vi "Autonomous Independent.vi"() -> ()   [LabVIEW 2013]
doc: "This VI is called when autonomous begins, and will automatically be terminated when autonomous ends. You can carry out timed or sensor driven robot movement independently without needing to return to the caller."
uses:
  <vilib>/Rock Robotics/WPI/Solenoid/WPI_SolenoidValue.ctl
  Robot Global Data.vi
  <vilib>/Rock Robotics/WPI/Solenoid/WPI_SolenoidSetEnum.vi
  <vilib>/Rock Robotics/WPI/RobotDrive/WPI_RobotDriveArcadeDrive_Standard(NoSaturation).vi
  <vilib>/Rock Robotics/WPI/RobotDrive/WPI_RobotDriveGetSetRefNum.vi
  <vilib>/Rock Robotics/WPI/Joystick/WPI_JoystickGetSetRefNum.vi
panel:
  out "Motor Values":dbl[](array[numeric])
  in  "Current Shooter Status":T1(ring)
  out "Timer for firing mech 2":dbl
  out "Timer for firing mech":dbl
  out "Hot?":bool
  out "Current Movement, for debugging":T2 {"Y Joystick Value" scale=1.0..-1.0; "X Joystick Value" scale=-1.0..1.0}
  in  "Array of robot movements":T3(array[cluster]) {"Y Joystick Value" scale=1.0..-1.0; "X Joystick Value" scale=-1.0..1.0}
  # "Be sure to right-click and choose Data Operations>>Make Current Value default if you want to save the array values with the VI"
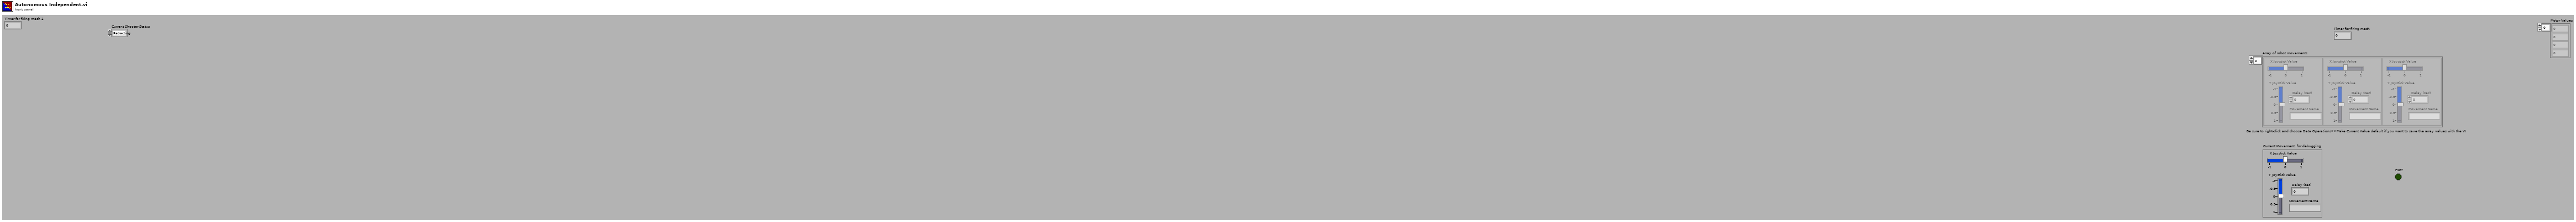
[diagram p1: front panel]
types:
  T1 = enum16{"Retracting", "Firing", "Ready to fire", "Pulling back", "Just fired"}
  T2 = cluster{"X Joystick Value":dbl, "Y Joystick Value":dbl, "Delay (sec)":dbl, "Movement Name":string}
  T3 = cluster{"X Joystick Value":dbl, "Y Joystick Value":dbl, "Delay (sec)":dbl, "Movement Name":string}[]
  T4 = typedef "WPI_JoystickDevRef.ctl" = cluster{"Device":T5}
  T5 = typedef "WPI_JoystickDeviceEnum.ctl" = enum16{"USB 1", "USB 2", "USB 3", "USB 4", "Kinect 1", "Kinect 2"}
  T6 = cluster{"axis 1 (x)":dbl, "axis 2 (y)":dbl, "axis 3 (throttle)":dbl, "axis 4":dbl, "axis 5":dbl, "axis 6":dbl}
  T7 = typedef "WPI_MotorControlDeviceRef.ctl" = cluster{"DeviceStatus":errorcluster, "Type":enum16{"PWM", "CAN"}, "PWM":cluster{"Digital Module":T8, "PWM Channel":T9, "DeadBand":T10}, "CAN":cluster{"Device Number":u8, "Control Mode":T11, "Semaphore":T12, "Max Vout":dbl}, "Invert":bool, "TransformRef":T13, "InvTransformRef":T13}
  T8 = typedef "FPGA_TypedefDigitalModule.ctl" = enum16{"Digital Module 1", "Digital Module 2"}
  T9 = typedef "FPGA_DIOPWMChannel.ctl" = enum8{"PWM 1", "PWM 2", "PWM 3", "PWM 4", "PWM 5", "PWM 6", "PWM 7", "PWM 8", "PWM 9", "PWM 10", "Invalid"}
  T10 = typedef "WPI_PWMDeadband.ctl" = cluster{"Name":string, "maxPositivePwm":i32, "minPositivePwm":i32, "centerPwm":i32, "maxNegativePwm":i32, "minNegativePwm":i32, "angularRange":u16}
  T11 = typedef "WPI_CANJaguar_ControlMode.ctl" = enum8{"Percent VBus", "Current", "Speed", "Position", "Voltage"}
  T12 = typedef "Semaphore RefNum" = refnum<k1>
  T13 = typedef "WPI_PWMTransform_ConPane.ctl" = refnum<vi>
  T14 = typedef "WPI_RobotDriveDevRef.ctl" = cluster{"DevStatus":errorcluster, "Motors[]":T7[], "Square Inputs":bool, "Max Output":dbl, "Isochronous":bool}
  T15 = typedef "WPI_EncoderDevRef.ctl" = cluster{"DevStatus":errorcluster, "EncoderIndex":T16, "CounterIndex":T17, "DistancePerCount":dbl, "Decoding Type":T18}
  T16 = typedef "FPGA_EncoderIdx.ctl" = enum8{"Enc 0", "Enc 1", "Enc 2", "Enc 3", "Invalid"}
  T17 = typedef "FPGA_CounterCtrSystemIndex.ctl" = enum8{"Ctr 0", "Ctr 1", "Ctr 2", "Ctr 3", "Ctr 4", "Ctr 5", "Ctr 6", "Ctr 7", "Invalid"}
  T18 = typedef "WPI_EncoderType.ctl" = enum16{"1x", "2x", "4x"}
  T19 = typedef "WPI_DigitalInputDevRef.ctl" = cluster{"DevStatus":errorcluster, "DIO Channel":T20, "Digital Module":T8}
  T20 = typedef "FPGA_DIOChannel.ctl" = enum8{"DIO 1", "DIO 2", "DIO 3", "DIO 4", "DIO 5", "DIO 6", "DIO 7", "DIO 8", "DIO 9", "DIO 10", "DIO 11", "DIO 12", "DIO 13", "DIO 14", "Invalid"}
  T21 = typedef "WPI_SolenoidValue.ctl" = enum16{"Off", "On", "Forward", "Reverse"}
  T22 = typedef "WPI_SolenoidDevRef.ctl" = cluster{"DevStatus":errorcluster, "Solenoid Module":T23, "Forward Solenoid Channel":T24, "Reverse Solenoid Channel":T24}
  T23 = typedef "FPGA_TypedefSolenoidModule.ctl" = enum16{"Solenoid Module 1", "Solenoid Module 2"}
  T24 = typedef "WPI_SolenoidChannel.ctl" = enum8{"Solenoid 1", "Solenoid 2", "Solenoid 3", "Solenoid 4", "Solenoid 5", "Solenoid 6", "Solenoid 7", "Solenoid 8", "Invalid"}
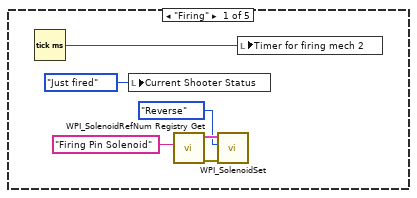
[diagram p2: hidden frame]
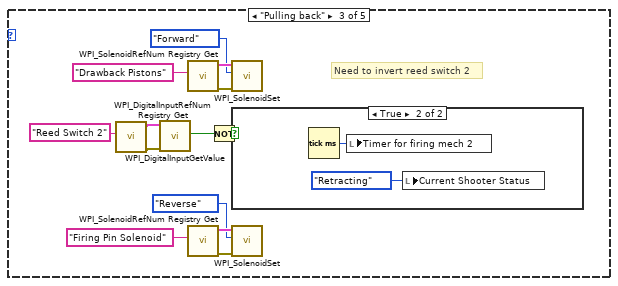
[diagram p3: hidden frame]
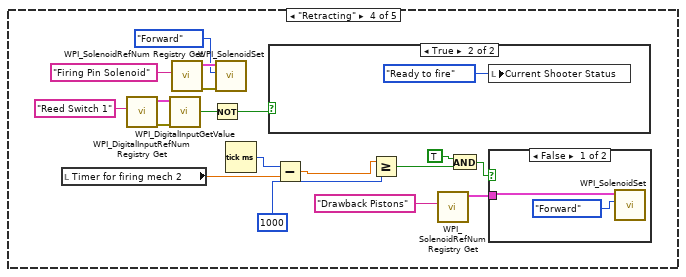
[diagram p5: hidden frame]
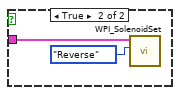
[diagram p7: hidden frame]
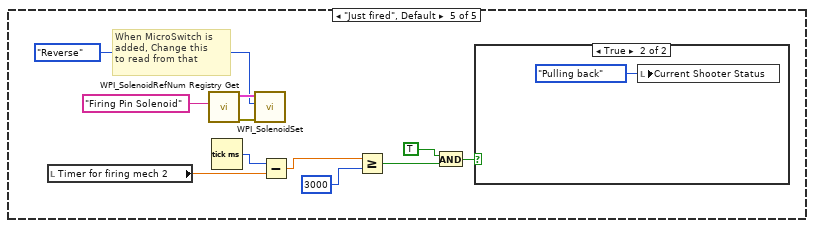
[diagram p8: hidden frame]
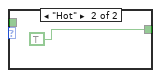
[diagram p14: hidden frame]
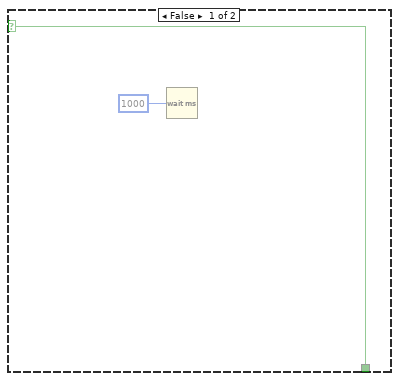
[diagram p15: hidden frame]
diagram:
  (unwired) "This code sets the toggle rate used by the Periodic Tasks VI.  For autonomous mode we slowly flash the USER1 LED on the cRIO.  Look at the Periodic Tasks VI to see how this global value is used."
  (unwired) "Autonomous sample code is disabled so your robot doesn't unexpectantly run in Autonomous mode.  To enable this code, right-click on the edge of the frame and choose either \"Remove Diagram Disable Structure\" or \"Enable This Subdiagram\". You should only enable one of the samples."
  (unwired) "This function is run in parallel when the autonomous period begins. It will be terminated automatically when the period ends.\n\nNote that all Driver Station inputs are automatically latched and will not change once auto begins."
  # "Every 20ms, report that we are running autonomous\ncode. Loop will abort the same time as the VI."
  # "This gives you the joystick value\nthat is often the throttle"
  # "Use time and/or sensors to control how the robot drives."
  # "This tells you the driver position\nand alliance color"
  # "This gives you the eight Driver Station\ndigital switch settings"
  # "This gives you the four\nDriver Station sliders or\nanalog voltages"
  n1 = while {
    stop <- FALSE stop-if-true
    n2 = call <vilib>:"WPI_DriverStationReport Robot Code State.vi"("Autonomous"=TRUE) -> ()  [unwired: 10 in, 1 out]
    n3 = Wait (ms)(milliseconds to wait=u32 20) -> ()  [unwired: 1 out]
  }
  n4 = call <vilib>:"WPI_DriverStationGet Alliance Info.vi"() -> ()  [unwired: 12 out]
  n5 = call <vilib>:"WPI_DriverStationGet Digital Input.vi"() -> ("Driver Station Digital Input (1-8)"=w13:bool[])  [unwired: 11 out]
  n6 = call <vilib>:"WPI_DriverStationGet Analog Input.vi"() -> ()  [unwired: 12 out]
  n7 = global write "Robot Global Data.vi" "LED toggle rate (ms)"(u32 500 ("LED ms toggle rate")) -> ()
  n8 = call <vilib>:"WPI_JoystickRefNum Registry Get.vi"("refnum name"="Joystick 1") -> ("JoystickDevRef"=w11:T4)  [unwired: 1 in, 9 out]
  n9 = call <vilib>:"WPI_JoystickGet.vi"("JoystickDevRef"=w11) -> ("Axes"=w8:T6)  [unwired: 1 in, 5 out]
  n10 = Cluster To Array(cluster=w8) -> (array=w9:dbl[])
  n11 = Unbundle By Name(w8) -> ()  [unwired: 1 out]
  n12 = call <vilib>:"SD Write Numeric Array.vi"("Numeric Array"=w9, "Name"="Joystick 1/Axes") -> ()  [unwired: 8 in, 2 out]
  n13 = Index Array(array=w13) -> ()  [unwired: 8 in, 8 out]
  n14 = disable-structure shown="Disabled" {
    frame Disabled {
      w17 = "RobotDrive Motors" ("Name")
      # "This is some simple sample code to drive your robot curving one direction and then the other."
      # "stand still"
      # "turn left for 0.5 second"
      # "turn right for 1 second"
      n15 = while {
        stop <- w38 stop-if-true
        n16 = call "2014 Target Detection.vi"() -> (2:w37)  [unwired: 11 in]
        n17 = for {
          tunnel: w37 -> [w43] mode=indexing
          tunnel: [w42] -> _ mode=indexing
          shift-right: [w40] -> w35
          shift-left: FALSE -> [w39]
          n18 = Unbundle By Name(w43) -> ("Scores"=w42)  [unwired: 4 out]
          n19 = Unbundle By Name(w42) -> ("State"=w41)
          n20 = case shown="\"Not Hot\", Default" w41 {
            tunnel: [w44 TRUE] -> w40
            tunnel: w39 -> [w44 _]
            frame "Not Hot", Default {
            }
            frame "Hot" {
            }
          }
        }
        n21 = case shown="True" w35 {
          selector: w35 -> [w46 _]
          tunnel: [w46 w48] -> w38
          frame False {
            n22 = Wait (ms)(milliseconds to wait=1000) -> ()  [unwired: 1 out]
          }
          frame True {
            w48 = TRUE
            n23 = flat-sequence {
              frame #0 {
                n24 = call <vilib>:"WPI_MotorControlRefNum Registry Get.vi"("refnum name"="Mechanism Motor 1") -> ("MotorControlDevRef"=w52:T7)  [unwired: 9 in, 1 out]
                n25 = call <vilib>:"WPI_MotorControlSetOutput.vi"("Output"=0.5, "MotorControlDevRef"=w52) -> ("MotorControlDevRef"=w50:T7)  [unwired: 7 in, 2 out]
                n26 = Wait (ms)(milliseconds to wait=2000) -> ()  [unwired: 1 out]
                n27 = call <vilib>:"WPI_MotorControlGetOutput.vi"("MotorControlDevRef"=w50) -> ()  [unwired: 8 in, 3 out]
              }
              frame #1 {
                n28 = call <vilib>:"WPI_MotorControlRefNum Registry Get.vi"("refnum name"="Mechanism Motor 1") -> ("MotorControlDevRef"=w56:T7)  [unwired: 9 in, 1 out]
                n29 = call <vilib>:"WPI_MotorControlSetOutput.vi"("Output"=0.0, "MotorControlDevRef"=w56) -> ("MotorControlDevRef"=w54:T7)  [unwired: 7 in, 2 out]
                n30 = call <vilib>:"WPI_MotorControlGetOutput.vi"("MotorControlDevRef"=w54) -> ()  [unwired: 8 in, 3 out]
              }
            }
            "Hot?" <- w48
          }
        }
      }
      n31 = call <vilib>:"WPI_RobotDriveRefNum Registry Get.vi"("refnum name"="Left and Right Motors") -> ("RobotDriveDevRef"=w21:T14)  [unwired: 1 in, 9 out]
      n32 = call-poly <vilib>:"WPI_RobotDriveArcadeDrive.vi"("Y axis value"=0.0 ("X axis value"), "X axis value"=0.0, "RobotDriveDevRef"=w21) -> ("Motor Values"=w20:dbl[], "RobotDriveDevRef"=w28:T14)  [unwired: 1 in, 6 out]
      n33 = call <vilib>:"SD Write Numeric Array.vi"("Numeric Array"=w20, "Name"=w17) -> ()  [unwired: 8 in, 2 out]
      n34 = call <vilib>:"WPI_RobotDriveDelayAndUpdateSafety.vi"("Delay (s)"=0.0, "RobotDriveDevRef"=w28) -> ("RobotDriveDevRef 2"=w27:T14)  [unwired: 8 in, 1 out]
      n35 = call-poly <vilib>:"WPI_RobotDriveArcadeDrive.vi"("Y axis value"=0.0 ("X axis value"), "X axis value"=0.0, "RobotDriveDevRef"=w27) -> ("Motor Values"=w19:dbl[], "RobotDriveDevRef"=w26:T14)  [unwired: 1 in, 6 out]
      n36 = call <vilib>:"SD Write Numeric Array.vi"("Numeric Array"=w19, "Name"=w17) -> ()  [unwired: 8 in, 2 out]
      n37 = call <vilib>:"WPI_RobotDriveDelayAndUpdateSafety.vi"("Delay (s)"=0.0, "RobotDriveDevRef"=w26) -> ("RobotDriveDevRef 2"=w25:T14)  [unwired: 8 in, 1 out]
      n38 = call-poly <vilib>:"WPI_RobotDriveArcadeDrive.vi"("Y axis value"=0.0 ("X axis value"), "X axis value"=0.0, "RobotDriveDevRef"=w25) -> ("Motor Values"=w18:dbl[])  [unwired: 1 in, 7 out]
      n39 = call <vilib>:"SD Write Numeric Array.vi"("Numeric Array"=w18, "Name"=w17) -> ()  [unwired: 8 in, 2 out]
    }
    frame Disabled {
    }
    frame Enabled {
    }
  }
  n40 = disable-structure shown="Disabled" {
    frame Disabled {
      # "This sample code describes robot movements in an array. You can extend it to control other motors\non your robot. You can also use file I/O to move the data to a text file."
      n41 = call <vilib>:"WPI_RobotDriveRefNum Registry Get.vi"("refnum name"="Left and Right Motors") -> ("RobotDriveDevRef"=w59:T14)  [unwired: 1 in, 9 out]
      n42 = for {
        shift-right: [w65] -> _
        shift-left: w59 -> [w66]
        tunnel: "Array of robot movements" -> [w61] mode=indexing
        n43 = Unbundle By Name(w61) -> ("X Joystick Value"=w64:dbl, "Y Joystick Value"=w63:dbl, "Delay (sec)"=w62:dbl)  [unwired: 1 out]
        n44 = call-poly <vilib>:"WPI_RobotDriveArcadeDrive.vi"("Y axis value"=w63, "X axis value"=w64, "RobotDriveDevRef"=w66) -> ("Motor Values"=w68:dbl[], "RobotDriveDevRef"=w67:T14)  [unwired: 1 in, 6 out]
        n45 = call <vilib>:"SD Write Numeric Array.vi"("Numeric Array"=w68, "Name"="RobotDrive Motors") -> ()  [unwired: 8 in, 2 out]
        n46 = call <vilib>:"WPI_RobotDriveDelayAndUpdateSafety.vi"("Delay (s)"=w62, "RobotDriveDevRef"=w67) -> ("RobotDriveDevRef 2"=w65:T14)  [unwired: 8 in, 1 out]
        "Current Movement, for debugging" <- w61
      }
    }
    frame Enabled {
    }
  }
  n47 = flat-sequence {
    tunnel: [TRUE] -> w3
    frame #0 {
      # "CHECK REFNUM"
      n48 = disable-structure shown="Disabled" {
        frame Disabled {
          n49 = Tick Count (ms)() -> (millisecond timer value=w76:u32)
          n50 = while {
            tunnel: w76 -> [w81]
            stop <- w78 stop-if-true
            n51 = call <vilib>:"WPI_RobotDriveRefNum Registry Get.vi"("refnum name"="Left and Right Motors") -> ("error out"=w87:errorcluster, "RobotDriveDevRef"=w86:T14)  [unwired: 9 in]
            n52 = call-poly <vilib>:"WPI_RobotDriveArcadeDrive.vi"("error in (no error)"=w87, "Y axis value"=-0.8, "X axis value"=0.1, "RobotDriveDevRef"=w86) -> ("Motor Values"=→"Motor Values":dbl[])  [unwired: 5 in, 2 out]
            n53 = Tick Count (ms)() -> (millisecond timer value=w82:u32)
            n54 = Subtract(x=w82, y=w81) -> (x-y=w80:u32)
            n55 = Greater?(x=w80, y=u32 5000) -> (0:w78:bool)
          }
        }
        frame Enabled {
        }
      }
      n56 = call <vilib>:"WPI_EncoderRefNum Registry Get.vi"("refnum name"="Right Drive Encoder") -> ("error out"=w75:errorcluster, "EncoderDevRef"=w74:T15)  [unwired: 9 in]
      n57 = call <vilib>:"WPI_EncoderReset.vi"("error in (no error)"=w75, "EncoderDevRef"=w74) -> ()  [unwired: 8 in, 2 out]
      n58 = call <vilib>:"WPI_EncoderRefNum Registry Get.vi"("refnum name"="Left Drive Encoder") -> ("error out"=w72:errorcluster, "EncoderDevRef"=w71:T15)  [unwired: 9 in]
      n59 = call <vilib>:"WPI_EncoderReset.vi"("error in (no error)"=w72, "EncoderDevRef"=w71) -> ()  [unwired: 8 in, 2 out]
    }
    frame #1 {
      n60 = while {
        stop <- w88 stop-if-true
        n61 = call "distancepidinit.vi"("Distance From Target"=18.5) -> ("Done?"=w88:bool)  [unwired: 10 in]
      }
    }
    frame #2 {
      n62 = call <vilib>:"WPI_RobotDriveRefNum Registry Get.vi"("refnum name"="Left and Right Motors") -> ("error out"=w95:errorcluster, "RobotDriveDevRef"=w94:T14)  [unwired: 9 in]
      n63 = call-poly <vilib>:"WPI_RobotDriveArcadeDrive.vi"("error in (no error)"=w95, "Y axis value"=0.0, "X axis value"=0.0, "RobotDriveDevRef"=w94) -> ()  [unwired: 5 in, 3 out]
    }
  }
  n64 = flat-sequence {
    tunnel: [w96] -> w6
    tunnel: w6 -> [w107]
    tunnel: [TRUE] -> w2
    frame #0 {
      n65 = while {
        tunnel: [w101] -> w96
        stop <- w97 stop-if-true
        n66 = call <vilib>:"WPI_DigitalInputRefNum Registry Get.vi"("refnum name"="Top Limit Switch") -> ("error out"=w98:errorcluster, "DigitalInputDevRef"=w99:T19)  [unwired: 9 in]
        n67 = call <vilib>:"WPI_DigitalInputGetValue.vi"("error in (no error)"=w98, "DigitalInputDevRef"=w99) -> ("Value"=w97:bool)  [unwired: 7 in, 2 out]
        n68 = call <vilib>:"WPI_MotorControlRefNum Registry Get.vi"("refnum name"="Fisher Price") -> ("error out"=w104:errorcluster, "MotorControlDevRef"=w103:T7)  [unwired: 9 in]
        n69 = call <vilib>:"WPI_MotorControlSetOutput.vi"("error in (no error)"=w104, "Output"=-0.2, "MotorControlDevRef"=w103) -> ("MotorControlDevRef"=w101:T7)  [unwired: 6 in, 2 out]
      }
    }
    frame #1 {
      n70 = call <vilib>:"WPI_MotorControlSetOutput.vi"("Output"=0.0, "MotorControlDevRef"=w107) -> ()  [unwired: 7 in, 3 out]
    }
  }
  n71 = disable-structure shown="Disabled" {
    frame Disabled {
      n72 = call <vilib>:"WPI_MotorControlRefNum Registry Get.vi"("refnum name"="Mechanism Motor 2") -> ("MotorControlDevRef"=w116:T7)  [unwired: 9 in, 1 out]
      n73 = call <vilib>:"WPI_MotorControlRefNum Registry Get.vi"("refnum name"="Mechanism Motor 3") -> ("MotorControlDevRef"=w111:T7)  [unwired: 9 in, 1 out]
      n74 = call <vilib>:"WPI_MotorControlSetOutput.vi"("Output"=0.5, "MotorControlDevRef"=w116) -> ("MotorControlDevRef"=w114:T7)  [unwired: 7 in, 2 out]
      n75 = call <vilib>:"WPI_MotorControlSetOutput.vi"("Output"=0.5, "MotorControlDevRef"=w111) -> ("MotorControlDevRef"=w109:T7)  [unwired: 7 in, 2 out]
      n76 = call <vilib>:"WPI_MotorControlGetOutput.vi"("MotorControlDevRef"=w114) -> ()  [unwired: 8 in, 3 out]
      n77 = call <vilib>:"WPI_MotorControlGetOutput.vi"("MotorControlDevRef"=w109) -> ()  [unwired: 8 in, 3 out]
    }
    frame Enabled {
    }
  }
  n78 = while {
    stop <- FALSE stop-if-true
    n79 = case shown="\"Ready to fire\"" "Current Shooter Status" {
      frame "Firing" {
        n80 = Tick Count (ms)() -> (millisecond timer value=w120:u32)
        n81 = local write "Current Shooter Status"(T1."Just fired" ("Current Shooter Status")) -> ()
        n82 = call <vilib>:"WPI_SolenoidRefNum Registry Get.vi"("refnum name"="Firing Pin Solenoid") -> ("error out"=w124:errorcluster, "SolenoidDevRef"=w123:T22)  [unwired: 9 in]
        n83 = call-poly <vilib>:"WPI_SolenoidSet.vi"("error in (no error)"=w124, "Value"=WPI_SolenoidValue."Reverse", "SolenoidDevRef"=w123) -> ()  [unwired: 7 in, 2 out]
        n84 = local write "Timer for firing mech 2"(w120) -> ()
      }
      frame "Ready to fire" {
      }
      frame "Pulling back" {
        # "Need to invert reed switch 2"
        n85 = call <vilib>:"WPI_DigitalInputRefNum Registry Get.vi"("refnum name"="Reed Switch 2") -> ("error out"=w128:errorcluster, "DigitalInputDevRef"=w129:T19)  [unwired: 9 in]
        n86 = call <vilib>:"WPI_DigitalInputGetValue.vi"("error in (no error)"=w128, "DigitalInputDevRef"=w129) -> ("Value"=w127:bool)  [unwired: 7 in, 2 out]
        n87 = call <vilib>:"WPI_SolenoidRefNum Registry Get.vi"("refnum name"="Drawback Pistons") -> ("error out"=w133:errorcluster, "SolenoidDevRef"=w132:T22)  [unwired: 9 in]
        n88 = call <vilib>:"WPI_SolenoidRefNum Registry Get.vi"("refnum name"="Firing Pin Solenoid") -> ("error out"=w137:errorcluster, "SolenoidDevRef"=w136:T22)  [unwired: 9 in]
        n89 = Not(x=w127) -> (.not. x?=w126:bool)
        n90 = call-poly <vilib>:"WPI_SolenoidSet.vi"("error in (no error)"=w133, "Value"=WPI_SolenoidValue."Forward", "SolenoidDevRef"=w132) -> ()  [unwired: 7 in, 2 out]
        n91 = case shown="True" w126 {
          frame False {
          }
          frame True {
            n92 = Tick Count (ms)() -> (millisecond timer value=w139:u32)
            n93 = local write "Timer for firing mech 2"(w139) -> ()
            n94 = local write "Current Shooter Status"(T1."Retracting" ("Current Shooter Status")) -> ()
          }
        }
        n95 = call-poly <vilib>:"WPI_SolenoidSet.vi"("error in (no error)"=w137, "Value"=WPI_SolenoidValue."Reverse", "SolenoidDevRef"=w136) -> ()  [unwired: 7 in, 2 out]
      }
      frame "Retracting" {
        n96 = local read "Timer for firing mech 2"() -> (w154:dbl)
        n97 = call <vilib>:"WPI_DigitalInputRefNum Registry Get.vi"("refnum name"="Reed Switch 1") -> ("error out"=w148:errorcluster, "DigitalInputDevRef"=w149:T19)  [unwired: 9 in]
        n98 = call <vilib>:"WPI_DigitalInputGetValue.vi"("error in (no error)"=w148, "DigitalInputDevRef"=w149) -> ("Value"=w141:bool)  [unwired: 7 in, 2 out]
        n99 = call <vilib>:"WPI_SolenoidRefNum Registry Get.vi"("refnum name"="Firing Pin Solenoid") -> ("error out"=w157:errorcluster, "SolenoidDevRef"=w156:T22)  [unwired: 9 in]
        n100 = Not(x=w141) -> (.not. x?=w142:bool)
        n101 = call-poly <vilib>:"WPI_SolenoidSet.vi"("error in (no error)"=w157, "Value"=WPI_SolenoidValue."Forward", "SolenoidDevRef"=w156) -> ()  [unwired: 7 in, 2 out]
        n102 = Tick Count (ms)() -> (millisecond timer value=w153:u32)
        n103 = case shown="True" w142 {
          frame False {
          }
          frame True {
            n104 = local write "Current Shooter Status"(T1."Ready to fire" ("Current Shooter Status")) -> ()
          }
        }
        n105 = Subtract(x=w153, y=w154) -> (x-y=w144:dbl)
        n106 = Greater Or Equal?(x=w144, y=1000) -> (x >= y?=w146:bool)
        n107 = call <vilib>:"WPI_SolenoidRefNum Registry Get.vi"("refnum name"="Drawback Pistons") -> ("SolenoidDevRef"=w151:T22)  [unwired: 9 in, 1 out]
        n108 = And(x=TRUE, y=w146) -> (x .and. y?=w147:bool)
        n109 = case shown="False" w147 {
          tunnel: w151 -> [w160 w162]
          frame False {
            n110 = call-poly <vilib>:"WPI_SolenoidSet.vi"("Value"=WPI_SolenoidValue."Forward", "SolenoidDevRef"=w160) -> ()  [unwired: 8 in, 2 out]
          }
          frame True {
            n111 = call-poly <vilib>:"WPI_SolenoidSet.vi"("Value"=WPI_SolenoidValue."Reverse", "SolenoidDevRef"=w162) -> ()  [unwired: 8 in, 2 out]
          }
        }
      }
      frame "Just fired", Default {
        # "When MicroSwitch is \nadded, Change this \nto read from that"
        n112 = local read "Timer for firing mech 2"() -> (w174:dbl)
        n113 = call <vilib>:"WPI_SolenoidRefNum Registry Get.vi"("refnum name"="Firing Pin Solenoid") -> ("error out"=w171:errorcluster, "SolenoidDevRef"=w170:T22)  [unwired: 9 in]
        n114 = Tick Count (ms)() -> (millisecond timer value=w173:u32)
        n115 = call-poly <vilib>:"WPI_SolenoidSet.vi"("error in (no error)"=w171, "Value"=WPI_SolenoidValue."Reverse", "SolenoidDevRef"=w170) -> ()  [unwired: 7 in, 2 out]
        n116 = Subtract(x=w173, y=w174) -> (x-y=w165:dbl)
        n117 = Greater Or Equal?(x=w165, y=3000) -> (x >= y?=w168:bool)
        n118 = And(x=TRUE, y=w168) -> (x .and. y?=w167:bool)
        n119 = case shown="True" w167 {
          frame False {
          }
          frame True {
            n120 = local write "Current Shooter Status"(T1."Pulling back" ("Current Shooter Status")) -> ()
          }
        }
      }
    }
    n121 = Wait (ms)(milliseconds to wait=u32 50) -> ()  [unwired: 1 out]
  }
  n122 = local write "Current Shooter Status"(T1."Ready to fire" ("Current Shooter Status")) -> ()
  n123 = And(x=w3, y=w2) -> (x .and. y?=w5:bool)
  n124 = flat-sequence {
    tunnel: [w181] -> w4
    tunnel: w5 -> [w181]
    tunnel: w4 -> [w182]
    frame #0 {
      n125 = call <vilib>:"WPI_SolenoidRefNum Registry Get.vi"("refnum name"="Grabber Pistons Solenoid") -> ("error out"=w178:errorcluster, "SolenoidDevRef"=w177:T22)  [unwired: 9 in]
      n126 = Wait (ms)(milliseconds to wait=u32 500) -> ()  [unwired: 1 out]
      n127 = call-poly <vilib>:"WPI_SolenoidSet.vi"("error in (no error)"=w178, "Value"=WPI_SolenoidValue."Forward", "SolenoidDevRef"=w177) -> ()  [unwired: 7 in, 2 out]
    }
    frame #1 {
      n128 = case shown="True" w182 {
        frame False {
        }
        frame True {
          n129 = local write "Current Shooter Status"(T1."Firing" ("Current Shooter Status")) -> ()
        }
      }
    }
    frame #2 {
      n130 = while {
        stop <- FALSE stop-if-true
        n131 = call <vilib>:"WPI_RobotDriveRefNum Registry Get.vi"("refnum name"="Left and Right Motors") -> ("error out"=w189:errorcluster, "RobotDriveDevRef"=w188:T14)  [unwired: 9 in]
        n132 = call-poly <vilib>:"WPI_RobotDriveArcadeDrive.vi"("error in (no error)"=w189, "Y axis value"=0.0, "X axis value"=0.0, "RobotDriveDevRef"=w188) -> ()  [unwired: 5 in, 3 out]
      }
    }
  }
